vi "MarbleDispenserMk7.vi"() -> ()   [LabVIEW 2016]
uses:
  <vilib>/NXT/Block Support/NXT_InputPort.ctl
  <vilib>/NXT/Block Support/NXT_OutputPort.ctl
  <vilib>/NXT/LegoClasses/BrickReference/BrickReference.lvclass
  <vilib>/NXT/Subs/LVHSConnector.ctl
  <vilib>/NXT/NXTIO Xnodes/NXTIOXNode/NXTIO.xnode
  <vilib>/NXT/NXTIO Xnodes/AddressXNode/NXTIOAddress.xnode
  <vilib>/NXT/NXTIO Xnodes/NXTIONodeSubVIs/NXTStopMotors.vi
  <vilib>/NXT/NXTIO Xnodes/NXTIONodeSubVIs/NXTMotorRunDistance.vi
  <vilib>/NXT/Dual Mode Library/Waits/Wait_Num.vi
  <vilib>/NXT/Dual Mode Library/Sensors/EV3_Color_Color.vi
  <vilib>/NXT/Dual Mode Library/Sensors/Touch_Released.vi
  <vilib>/NXT/Dual Mode Library/Sensors/Touch_Pressed.vi
panel:
  out "Numeric 2":dbl
  out "Numeric":dbl
  out "Speed":dbl
  out "Color":string
  out "Distance":dbl
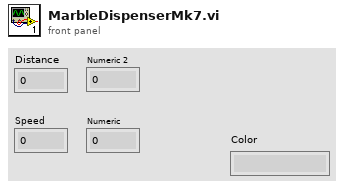
[diagram p1: front panel]
types:
  T1 = typedef "NXT_InputPort.ctl" = u32
  T2 = typedef "NXT_OutputPort.ctl" = u8
  T3 = typedef "LVHSConnector.ctl" = refnum<class "BrickReference.lvclass">
  T4 = typedef "ColorSensorColors.ctl" = enum16{"No Color", "Black", "Blue", "Green", "Yellow", "Red", "White", "Brown"}
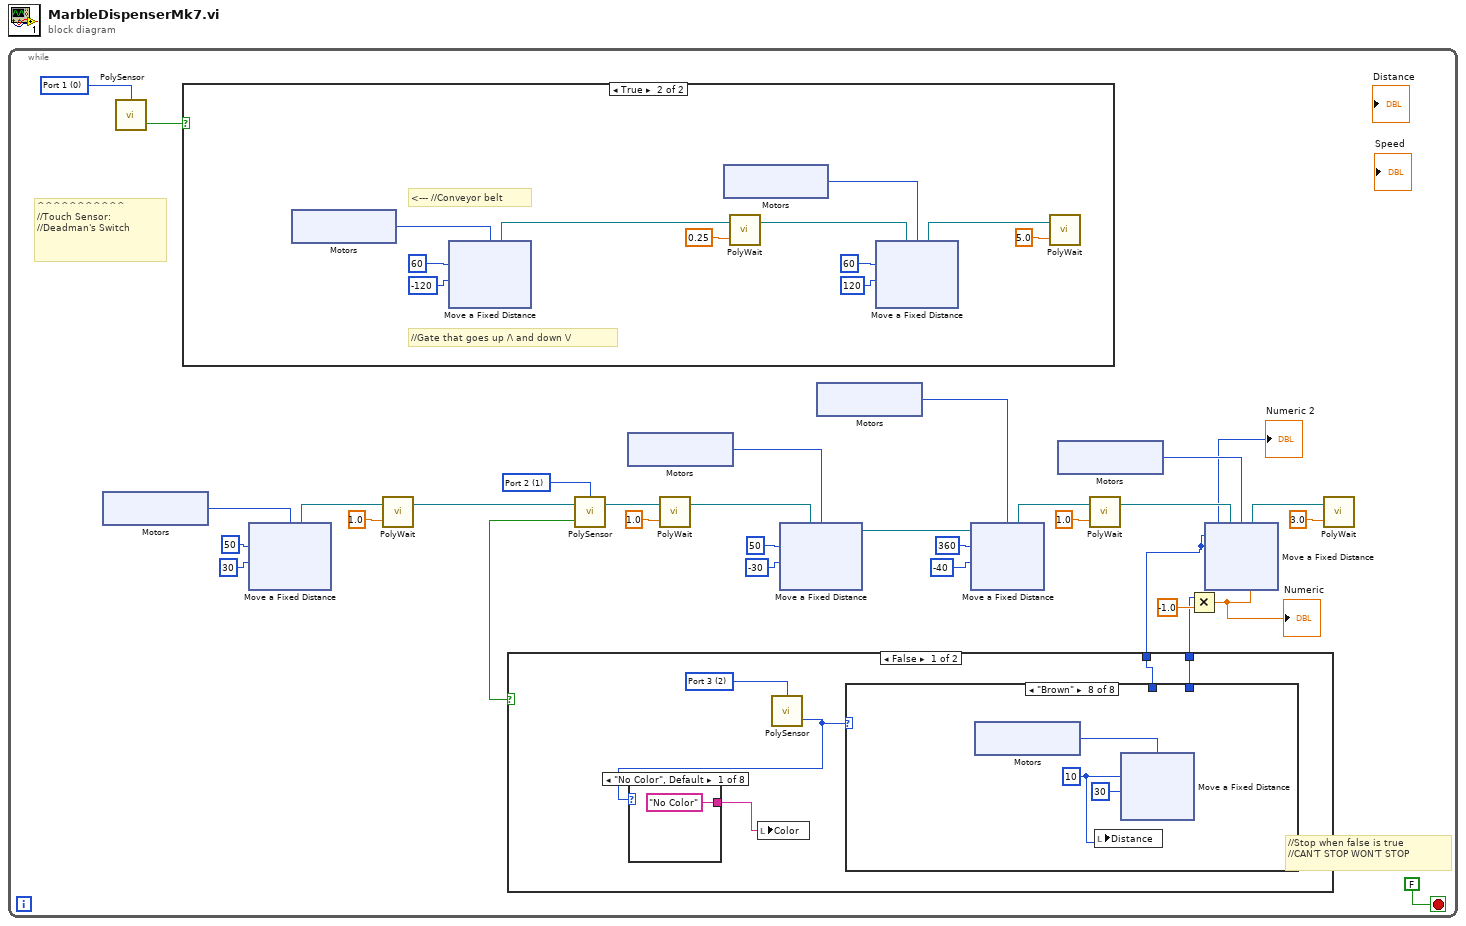
[diagram p0: block diagram]
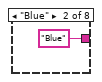
[diagram p2: hidden frame]
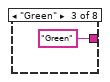
[diagram p3: hidden frame]
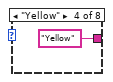
[diagram p4: hidden frame]
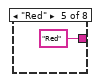
[diagram p5: hidden frame]
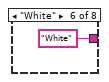
[diagram p6: hidden frame]
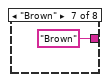
[diagram p7: hidden frame]
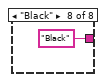
[diagram p8: hidden frame]
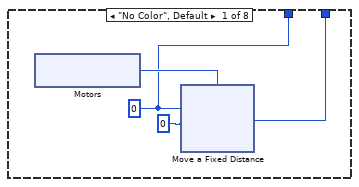
[diagram p9: hidden frame]
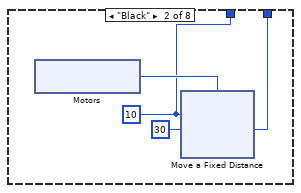
[diagram p10: hidden frame]
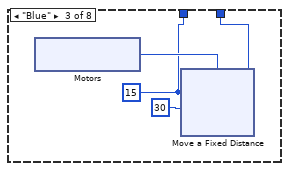
[diagram p11: hidden frame]
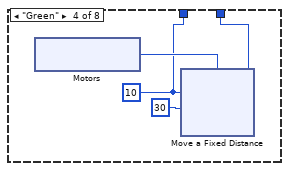
[diagram p12: hidden frame]
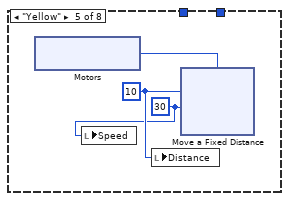
[diagram p13: hidden frame]
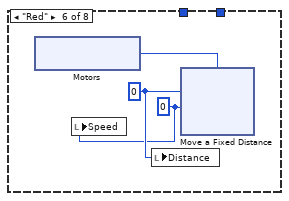
[diagram p14: hidden frame]
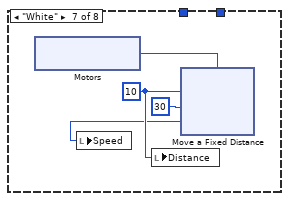
[diagram p15: hidden frame]
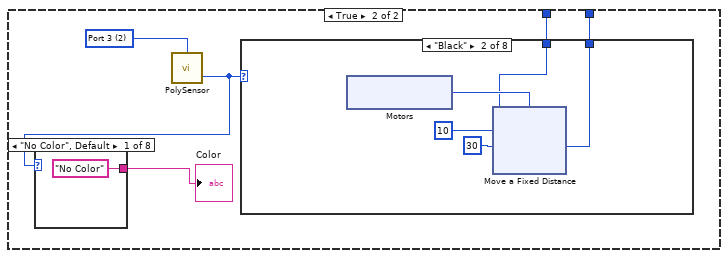
[diagram p16: hidden frame]
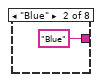
[diagram p17: hidden frame]
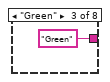
[diagram p18: hidden frame]
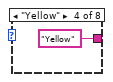
[diagram p19: hidden frame]
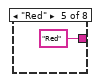
[diagram p20: hidden frame]
diagram:
  n1 = while {
    stop <- FALSE stop-if-true
    w18 = T1 1 items=["Port 1", "Port 2", "Port 3", "Port 4"] ("Port (Port 1)")
    w31 = T1 0 items=["Port 1", "Port 2", "Port 3", "Port 4"] ("Port (Port 1)")
    # "//Stop when false is true\n//CAN'T STOP WON'T STOP"
    # "^^^^^^^^^^^\n//Touch Sensor:\n//Deadman's Switch"
    n2 = xnode "Motors"() -> ("Motor"=w24:T2)
    n3 = call-poly <vilib>:"PolySensor.vi"("Port (Port 1)"=w31) -> ("Yes / No"=w29:bool)  [unwired: 2 in, 1 out]
    n4 = case shown="True" w29 {
      frame False {
        # "//This stops all the things"
        n5 = xnode "Motors"() -> ("Motor"=w327:T2)
        n6 = xnode "Motors"() -> ("Motor"=w326:T2)
        n7 = xnode "Stop Motors"("Motors"=w327) -> ()  [unwired: 1 in, 1 out]
        n8 = xnode "Stop Motors"("Motors"=w326) -> ()  [unwired: 1 in, 1 out]
      }
      frame True {
        # "//Gate that goes up /\\ and down \\/"
        # "<--- //Conveyor belt"
        n9 = xnode "Motors"() -> ("Motor"=w346:T2)
        n10 = xnode "Move a Fixed Distance"("Speed 1"=-120, "Distance 1"=60, "Motors"=w346) -> ("NXT/EV3"=w349:T3)  [unwired: 1 in]
        n11 = xnode "Motors"() -> ("Motor"=w340:T2)
        n12 = call-poly <vilib>:"PolyWait.vi"("Time (1 sec)"=0.25, "NXT/EV3"=w349) -> ("NXT/EV3"=w341:T3)  [unwired: 2 in]
        n13 = xnode "Move a Fixed Distance"("Speed 1"=120, "Distance 1"=60, "Motors"=w340, "NXT/EV3"=w341) -> ("NXT/EV3"=w344:T3)
        n14 = call-poly <vilib>:"PolyWait.vi"("Time (1 sec)"=5.0, "NXT/EV3"=w344) -> ()  [unwired: 2 in, 1 out]
      }
    }
    n15 = xnode "Move a Fixed Distance"("Speed 1"=30, "Distance 1"=50, "Motors"=w24) -> ("NXT/EV3"=w27:T3)  [unwired: 1 in]
    n16 = call-poly <vilib>:"PolyWait.vi"("Time (1 sec)"=1.0, "NXT/EV3"=w27) -> ("NXT/EV3"=w19:T3)  [unwired: 2 in]
    n17 = call-poly <vilib>:"PolySensor.vi"("NXT/EV3"=w19, "Port (Port 1)"=w18) -> ("Yes / No"=w17:bool, "NXT/EV3"=w16:T3)  [unwired: 1 in]
    n18 = case shown="False" w17 {
      tunnel: [w54 w180] -> w2
      tunnel: [w55 w179] -> w1
      frame False {
        w58 = T1 2 items=["Port 1", "Port 2", "Port 3", "Port 4"] ("Port (Port 1)")
        n19 = call-poly <vilib>:"PolySensor.vi"("Port (Port 1)"=w58) -> ("Detected Color"=w57:T4)  [unwired: 2 in, 1 out]
        n20 = case shown="\"No Color\", Default" w57 {
          tunnel: ["No Color" "Blue" "Green" "Yellow" "Red" "White" "Brown" "Black"] -> w56
          frame "No Color", Default {
          }
          frame "Blue" {
          }
          frame "Green" {
          }
          frame "Yellow" {
          }
          frame "Red" {
          }
          frame "White" {
          }
          frame "Brown" {
          }
          frame "Black" {
          }
        }
        n21 = local write "Color"(w56) -> ()
        n22 = case shown="\"Brown\"" w57 {
          tunnel: [w68 w82 w96 w110 _ _ _ _] -> w55
          tunnel: [w67 w81 w95 w109 _ _ _ _] -> w54
          frame "No Color", Default {
            w67 = i8 0 ("Speed 1")
            w68 = 0 ("Distance 1")
            n23 = xnode "Motors"() -> ("Motor"=w69:T2)
            n24 = xnode "Move a Fixed Distance"("Speed 1"=w67, "Distance 1"=w68, "Motors"=w69) -> ()  [unwired: 1 in, 1 out]
          }
          frame "Black" {
            w81 = i8 30 ("Speed 1")
            w82 = 10 ("Distance 1")
            n25 = xnode "Motors"() -> ("Motor"=w83:T2)
            n26 = xnode "Move a Fixed Distance"("Speed 1"=w81, "Distance 1"=w82, "Motors"=w83) -> ()  [unwired: 1 in, 1 out]
          }
          frame "Blue" {
            w95 = i8 30 ("Speed 1")
            w96 = 15 ("Distance 1")
            n27 = xnode "Motors"() -> ("Motor"=w97:T2)
            n28 = xnode "Move a Fixed Distance"("Speed 1"=w95, "Distance 1"=w96, "Motors"=w97) -> ()  [unwired: 1 in, 1 out]
          }
          frame "Green" {
            w109 = i8 30 ("Speed 1")
            w110 = 10 ("Distance 1")
            n29 = xnode "Motors"() -> ("Motor"=w111:T2)
            n30 = xnode "Move a Fixed Distance"("Speed 1"=w109, "Distance 1"=w110, "Motors"=w111) -> ()  [unwired: 1 in, 1 out]
          }
          frame "Yellow" {
            w123 = i8 30 ("Speed 1")
            w124 = 10 ("Distance 1")
            n31 = xnode "Motors"() -> ("Motor"=w125:T2)
            n32 = local write "Speed"(w123) -> ()
            n33 = local write "Distance"(w124) -> ()
            n34 = xnode "Move a Fixed Distance"("Speed 1"=w123, "Distance 1"=w124, "Motors"=w125) -> ()  [unwired: 1 in, 1 out]
          }
          frame "Red" {
            w137 = i8 0 ("Speed 1")
            w138 = 0 ("Distance 1")
            n35 = xnode "Motors"() -> ("Motor"=w139:T2)
            n36 = local write "Speed"(w137) -> ()
            n37 = local write "Distance"(w138) -> ()
            n38 = xnode "Move a Fixed Distance"("Speed 1"=w137, "Distance 1"=w138, "Motors"=w139) -> ()  [unwired: 1 in, 1 out]
          }
          frame "White" {
            w151 = i8 30 ("Speed 1")
            w152 = 10 ("Distance 1")
            n39 = xnode "Motors"() -> ("Motor"=w153:T2)
            n40 = local write "Speed"(w151) -> ()
            n41 = local write "Distance"(w152) -> ()
            n42 = xnode "Move a Fixed Distance"("Speed 1"=w151, "Distance 1"=w152, "Motors"=w153) -> ()  [unwired: 1 in, 1 out]
          }
          frame "Brown" {
            w166 = 10 ("Distance 1")
            n43 = xnode "Motors"() -> ("Motor"=w167:T2)
            n44 = local write "Distance"(w166) -> ()
            n45 = xnode "Move a Fixed Distance"("Speed 1"=i8 30, "Distance 1"=w166, "Motors"=w167) -> ()  [unwired: 1 in, 1 out]
          }
        }
      }
      frame True {
        w183 = T1 2 items=["Port 1", "Port 2", "Port 3", "Port 4"] ("Port (Port 1)")
        n46 = call-poly <vilib>:"PolySensor.vi"("Port (Port 1)"=w183) -> ("Detected Color"=w181:T4)  [unwired: 2 in, 1 out]
        n47 = case shown="\"No Color\", Default" w181 {
          tunnel: ["No Color" "Blue" "Green" "Yellow" "Red" "White" "Brown" "Black"] -> w182
          frame "No Color", Default {
          }
          frame "Blue" {
          }
          frame "Green" {
          }
          frame "Yellow" {
          }
          frame "Red" {
          }
          frame "White" {
          }
          frame "Brown" {
          }
          frame "Black" {
          }
        }
        "Color" <- w182
        n48 = case shown="\"Black\"" w181 {
          tunnel: [w192 w206 w221 w234 w248 w262 w276 w290] -> w180
          tunnel: [w193 w207 w220 w235 w249 w263 w277 w291] -> w179
          frame "No Color", Default {
            w192 = i8 0 ("Speed 1")
            w193 = 0 ("Distance 1")
            n49 = xnode "Motors"() -> ("Motor"=w194:T2)
            n50 = xnode "Move a Fixed Distance"("Speed 1"=w192, "Distance 1"=w193, "Motors"=w194) -> ()  [unwired: 1 in, 1 out]
          }
          frame "Black" {
            w206 = i8 30 ("Speed 1")
            w207 = 10 ("Distance 1")
            n51 = xnode "Motors"() -> ("Motor"=w208:T2)
            n52 = xnode "Move a Fixed Distance"("Speed 1"=w206, "Distance 1"=w207, "Motors"=w208) -> ()  [unwired: 1 in, 1 out]
          }
          frame "Blue" {
            w221 = i8 30 ("Speed 1")
            w220 = 20 ("Distance 1")
            n53 = xnode "Motors"() -> ("Motor"=w222:T2)
            n54 = xnode "Move a Fixed Distance"("Speed 1"=w221, "Distance 1"=w220, "Motors"=w222) -> ()  [unwired: 1 in, 1 out]
          }
          frame "Green" {
            w234 = i8 30 ("Speed 1")
            w235 = 10 ("Distance 1")
            n55 = xnode "Motors"() -> ("Motor"=w236:T2)
            n56 = xnode "Move a Fixed Distance"("Speed 1"=w234, "Distance 1"=w235, "Motors"=w236) -> ()  [unwired: 1 in, 1 out]
          }
          frame "Yellow" {
            w248 = i8 30 ("Speed 1")
            w249 = 10 ("Distance 1")
            n57 = xnode "Motors"() -> ("Motor"=w250:T2)
            n58 = xnode "Move a Fixed Distance"("Speed 1"=w248, "Distance 1"=w249, "Motors"=w250) -> ()  [unwired: 1 in, 1 out]
          }
          frame "Red" {
            w262 = i8 30 ("Speed 1")
            w263 = 10 ("Distance 1")
            n59 = xnode "Motors"() -> ("Motor"=w264:T2)
            n60 = xnode "Move a Fixed Distance"("Speed 1"=w262, "Distance 1"=w263, "Motors"=w264) -> ()  [unwired: 1 in, 1 out]
          }
          frame "White" {
            w276 = i8 30 ("Speed 1")
            w277 = 10 ("Distance 1")
            n61 = xnode "Motors"() -> ("Motor"=w278:T2)
            n62 = xnode "Move a Fixed Distance"("Speed 1"=w276, "Distance 1"=w277, "Motors"=w278) -> ()  [unwired: 1 in, 1 out]
          }
          frame "Brown" {
            w290 = i8 30 ("Speed 1")
            w291 = 10 ("Distance 1")
            n63 = xnode "Motors"() -> ("Motor"=w292:T2)
            n64 = xnode "Move a Fixed Distance"("Speed 1"=w290, "Distance 1"=w291, "Motors"=w292) -> ()  [unwired: 1 in, 1 out]
          }
        }
      }
    }
    "Numeric 2" <- w1
    n65 = xnode "Motors"() -> ("Motor"=w20:T2)
    n66 = call-poly <vilib>:"PolyWait.vi"("Time (1 sec)"=sgl 1.0, "NXT/EV3"=w16) -> ("NXT/EV3"=w15:T3)  [unwired: 2 in]
    n67 = xnode "Move a Fixed Distance"("Speed 1"=-30, "Distance 1"=50, "Motors"=w20, "NXT/EV3"=w15) -> ("NXT/EV3"=w5:T3)
    n68 = xnode "Motors"() -> ("Motor"=w12:T2)
    n69 = xnode "Move a Fixed Distance"("Speed 1"=i8 -40, "Distance 1"=360, "Motors"=w12, "NXT/EV3"=w5) -> ("NXT/EV3"=w13:T3)
    n70 = xnode "Motors"() -> ("Motor"=w7:T2)
    n71 = call-poly <vilib>:"PolyWait.vi"("Time (1 sec)"=1.0, "NXT/EV3"=w13) -> ("NXT/EV3"=w8:T3)  [unwired: 2 in]
    n72 = Multiply(x=w2, y=-1.0) -> (x*y=w3:dbl)
    "Numeric" <- w3
    n73 = xnode "Move a Fixed Distance"("Speed 1"=w3, "Distance 1"=w1, "Motors"=w7, "NXT/EV3"=w8) -> ("NXT/EV3"=w6:T3)
    n74 = call-poly <vilib>:"PolyWait.vi"("Time (1 sec)"=3.0, "NXT/EV3"=w6) -> ()  [unwired: 2 in, 1 out]
  }
